vi "Read Transceiver Response.vi"(8 "error in (no error)":errorcluster, 9 "timeout in ms (0)":i32, 11 "Plugin Interface in":refnum<class "Plugin Interface.lvclass">) -> (0 "error out":errorcluster, 1 "empty?":bool, 2 "response":T1, 3 "Plugin Interface out":refnum<class "Plugin Interface.lvclass">, 4 "# elements":u32)   [LabVIEW 2017, in "DSF Core.lvlib" / "Plugin Interface.lvclass"]
uses:
  Plugin Interface.lvclass
  C:/Git/DSF/Data Sharing Framework/Source/Core/Engine/Classes/Interfaces/Interface/Interface.lvclass
  Response Data.ctl
  Response.ctl
  Response Parameters.ctl
  Interface/Interface.lvclass/Interface.ctl
  Debug/FIFO Flags/FIFO Flags.lvclass/FIFO Flags.ctl
  Interface/Get Debug Flags.vi
  Interface/Read RT FIFO(16B).vi
  Interface/Get Response FIFO.vi
  Debug/FIFO Flags/Get Infinite Timeouts.vi
  Interface/Errors.vi
  Interface/Response Timeout.vi
  Interface/Interface.lvclass
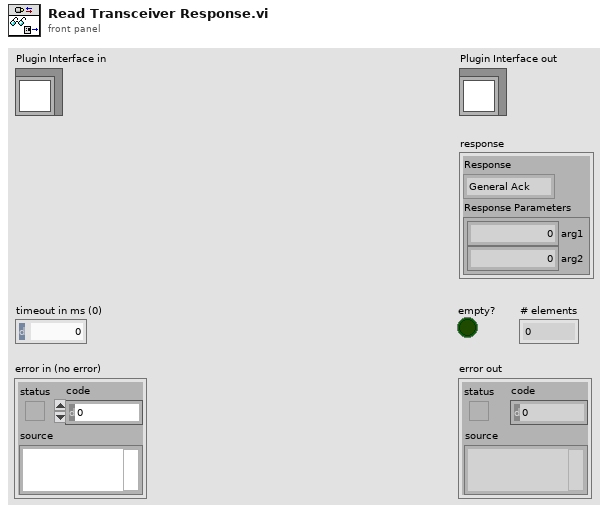
[diagram p1: front panel]
types:
  T1 = typedef "DSF Core.lvlib/Plugin Interface.lvclass/Response Data.ctl" = cluster{"Response":T2, "Response Parameters":T3}
  T2 = typedef "DSF Core.lvlib/Plugin Interface.lvclass/Response.ctl" = enum8{"General Ack", "Shutting Down"}
  T3 = typedef "DSF Core.lvlib/Plugin Interface.lvclass/Response Parameters.ctl" = cluster{"arg1":u64, "arg2":u64}
  T4 = typedef "DSF Core.lvlib/Interface.lvclass/RT FIFO Data 16B.ctl" = cluster{"Command":u8, "Payload":T5}
  T5 = typedef "DSF Core.lvlib/Interface.lvclass/RT FIFO Payload 16B.ctl" = cluster{"arg1":u64, "arg2":u64}
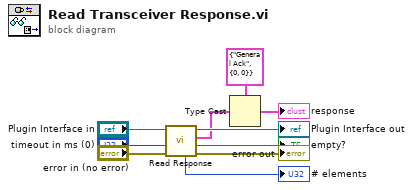
[diagram p0: block diagram]
diagram:
  n1 = call "Read Response.vi"("error in (no error)"="error in (no error)", "timeout in ms (0)"="timeout in ms (0)", "Interface in"="Plugin Interface in") -> ("error out"=→"error out":errorcluster, "timed out?"=→"empty?":bool, "response"=w6:T4, "Interface out"=→"Plugin Interface out":refnum<class "Plugin Interface.lvclass">, "# elements"=→"# elements":u32)  [unwired: 4 in]
  n2 = Type Cast(type=T1 {"Response"=enum."General Ack", "Response Parameters"={"arg1"=0, "arg2"=0}} ("Plugin Response"), x=w6) -> (*(type *) &x=→"response":T1)
